vi "Start Video.vi"(4 "AVI Path":path, 5 "Offset":cluster{"Ch1":u8, "Ch2":u8}, 6 "Save Movie?":bool, 7 "Gain(dB)":cluster{"Ch1":dbl, "Ch2":dbl}, 8 "error in":errorcluster, 9 "Frame Rate(Hz)":cluster{"AVI FR":i32, "Camera Fr":u16}={"AVI FR"=30, "Camera Fr"=0} {"AVI FR" min=2 max=3000 step=1}, 10 "Trigger Type":enum16{"Internal", "External"}(ring)=enum."External", 11 "Region of interest":i32[](array[numeric])) -> (0 "error out":errorcluster, 1 "Frame Buffers Out":T2[](array[typedef]), 2 "Avi Refnum":T1, 3 "IMAQ Session Out":refnum<k11>)   [LabVIEW 2013]
uses:
  <vilib>/vision/Image Controls.llb/IMAQ Image.ctl
  <vilib>/vision/Avi1.llb/AviRefnum.ctl
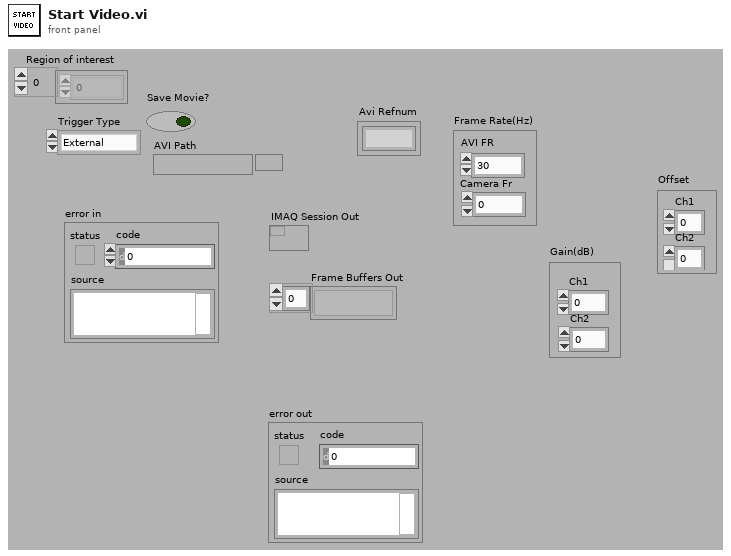
[diagram p1: front panel]
types:
  T1 = typedef "AviRefnum.ctl" = refnum<k1>
  T2 = typedef "IMAQ Image.ctl" = refnum<image>
  T3 = typedef "Image Type" = u32
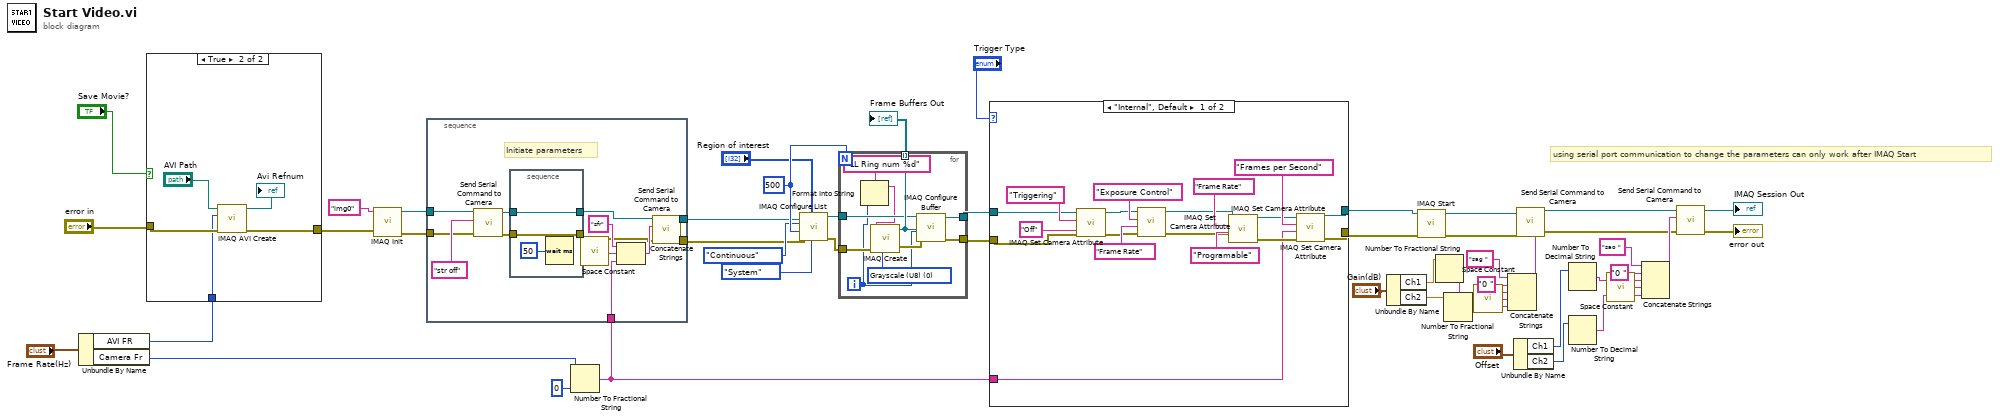
[diagram p0: block diagram]
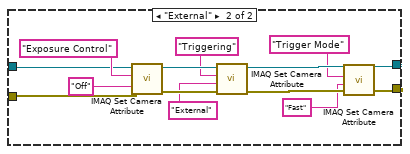
[diagram p3: hidden frame]
diagram:
  w49 = 500 ("Number of buffers")
  # "using serial port communication to change the parameters can only work after IMAQ Start"
  n1 = Unbundle By Name("Frame Rate(Hz)") -> ("AVI FR"=w27:i32, "Camera Fr"=w26:u16)
  n2 = case shown="True" "Save Movie?" {
    tunnel: "error in" -> [w50 w55]
    tunnel: [w50 w54] -> w40
    tunnel: w27 -> [_ w51]
    frame False {
    }
    frame True {
      n3 = call "IMAQ AVI Create"("error in (no error)"=w55, "Frames Per Second"=w51, "AVI Path"="AVI Path") -> ("error out"=w54:errorcluster, "Avi Refnum"=→"Avi Refnum":T1)  [unwired: 7 in]
    }
  }
  n4 = call <vilib>:"IMAQ Init.vi"("error in (no error)"=w40, "Interface Name"="img0") -> ("error out"=w35:errorcluster, "IMAQ Session Out"=w36:refnum<k11>)  [unwired: 8 in]
  n5 = Number To Fractional String(number=w26, precision (6)=i16 0) -> (F-format string=w31:string)  [unwired: 2 in]
  n6 = stacked-sequence {
    tunnel: w36 -> [w60]
    tunnel: w35 -> [w59]
    tunnel: [w58] -> w34
    tunnel: [w57] -> w33
    tunnel: w31 -> [w56]
    frame #0 {
      # "Initiate parameters"
      n7 = call "Send Serial Command to Camera.vi"("error in (no error)"=w59, "String to write"="str off", "IMAQ Session In"=w60) -> ("error out"=w62:errorcluster, "IMAQ Session Out"=w64:refnum<k11>)  [unwired: 5 in, 2 out]
      n8 = stacked-sequence {
        tunnel: w64 -> [w71]
        tunnel: [w71] -> w63
        tunnel: w62 -> [w70]
        tunnel: [w70] -> w61
        frame #0 {
          n9 = Wait (ms)(milliseconds to wait=u32 50) -> ()  [unwired: 1 out]
        }
      }
      n10 = call <vilib>:"Space Constant.vi"() -> ("String"=w66:string)
      n11 = Concatenate Strings("sfr" ("string"), w66, w56) -> (w65:string)
      n12 = call "Send Serial Command to Camera.vi"("error in (no error)"=w61, "String to write"=w65, "IMAQ Session In"=w63) -> ("error out"=w57:errorcluster, "IMAQ Session Out"=w58:refnum<k11>)  [unwired: 5 in, 2 out]
    }
  }
  n13 = call <vilib>:"IMAQ Configure List.vi"("Memory Location"=enum16{"System", "Onboard"}."System", "Region of interest"="Region of interest", "error in (no error)"=w33, "Number of buffers"=w49, "Continuous?"=enum16{"One-Shot", "Continuous"}."Continuous" ("Continuous ?"), "IMAQ Session In"=w34) -> ("error out"=w42:errorcluster, "IMAQ Session Out"=w43:refnum<k11>)  [unwired: 4 in]
  n14 = for {
    N: w49 -> [_]
    tunnel: [w81] -> w38
    tunnel: [w73] -> w37
    tunnel: w42 -> [w80]
    tunnel: w43 -> [w77]
    tunnel: [w78] -> w47 mode=indexing
    i -> [w74]
    w72 = T3 0 items=["Grayscale (U8)", "Grayscale (I16)", "Grayscale (SGL)", "Complex (CSG)", "RGB (U32)", "HSL (U32)", "RGB (U64)"] ("Image Type")
    n15 = Format Into String(format string="LL Ring num %d", w74) -> (resulting string=w76:string)  [unwired: 2 in, 1 out]
    n16 = call "IMAQ Create"("Image Name"=w76, "Image Type"=w72, "error in (no error)"=w80) -> ("New Image"=w78:T2, "error out"=w79:errorcluster)  [unwired: 2 in]
    n17 = call <vilib>:"IMAQ Configure Buffer.vi"("error in (no error)"=w79, "Buffer Number"=w74, "Image In"=w78, "IMAQ Session In"=w77) -> ("error out"=w73:errorcluster, "IMAQ Session Out"=w81:refnum<k11>)  [unwired: 6 in]
  }
  "Frame Buffers Out" <- w47
  n18 = case shown="\"Internal\", Default" "Trigger Type" {
    tunnel: w38 -> [w86 w103]
    tunnel: w37 -> [w85 w102]
    tunnel: w31 -> [w84 _]
    tunnel: [w83 w100] -> w30
    tunnel: [w82 w101] -> w29
    frame "Internal", Default {
      n19 = call <vilib>:"IMAQ Set Camera Attribute.vi"("error in (no error)"=w85, "Attribute Value"="Off", "Camera Attribute"="Triggering", "IMAQ Session In"=w86) -> ("error out"=w91:errorcluster, "IMAQ Session Out"=w93:refnum<k11>)  [unwired: 4 in]
      n20 = call <vilib>:"IMAQ Set Camera Attribute.vi"("error in (no error)"=w91, "Attribute Value"="Frame Rate", "Camera Attribute"="Exposure Control", "IMAQ Session In"=w93) -> ("error out"=w92:errorcluster, "IMAQ Session Out"=w94:refnum<k11>)  [unwired: 4 in]
      n21 = call <vilib>:"IMAQ Set Camera Attribute.vi"("error in (no error)"=w92, "Attribute Value"="Programable", "Camera Attribute"="Frame Rate", "IMAQ Session In"=w94) -> ("error out"=w90:errorcluster, "IMAQ Session Out"=w89:refnum<k11>)  [unwired: 4 in]
      n22 = call <vilib>:"IMAQ Set Camera Attribute.vi"("error in (no error)"=w90, "Attribute Value"=w84, "Camera Attribute"="Frames per Second", "IMAQ Session In"=w89) -> ("error out"=w82:errorcluster, "IMAQ Session Out"=w83:refnum<k11>)  [unwired: 4 in]
    }
    frame "External" {
      n23 = call <vilib>:"IMAQ Set Camera Attribute.vi"("error in (no error)"=w102, "Attribute Value"="Off", "Camera Attribute"="Exposure Control", "IMAQ Session In"=w103) -> ("error out"=w111:errorcluster, "IMAQ Session Out"=w109:refnum<k11>)  [unwired: 4 in]
      n24 = call <vilib>:"IMAQ Set Camera Attribute.vi"("error in (no error)"=w111, "Attribute Value"="External", "Camera Attribute"="Triggering", "IMAQ Session In"=w109) -> ("error out"=w110:errorcluster, "IMAQ Session Out"=w108:refnum<k11>)  [unwired: 4 in]
      n25 = call <vilib>:"IMAQ Set Camera Attribute.vi"("error in (no error)"=w110, "Attribute Value"="Fast", "Camera Attribute"="Trigger Mode", "IMAQ Session In"=w108) -> ("error out"=w101:errorcluster, "IMAQ Session Out"=w100:refnum<k11>)  [unwired: 4 in]
    }
  }
  n26 = Unbundle By Name("Gain(dB)") -> ("Ch1"=w15:dbl, "Ch2"=w14:dbl)
  n27 = call <vilib>:"IMAQ Start.vi"("error in (no error)"=w29, "IMAQ Session In"=w30) -> ("error out"=w16:errorcluster, "IMAQ Session Out"=w17:refnum<k11>)  [unwired: 8 in]
  n28 = Number To Fractional String(number=w15) -> (F-format string=w19:string)  [unwired: 3 in]
  n29 = Number To Fractional String(number=w14) -> (F-format string=w21:string)  [unwired: 3 in]
  n30 = call <vilib>:"Space Constant.vi"() -> ("String"=w20:string)
  n31 = Concatenate Strings("sag " ("String to write"), "0 " ("string"), w19, w20, w21) -> (w18:string)
  n32 = Unbundle By Name("Offset") -> ("Ch1"=w5:u8, "Ch2"=w4:u8)
  n33 = call "Send Serial Command to Camera.vi"("error in (no error)"=w16, "String to write"=w18, "IMAQ Session In"=w17) -> ("error out"=w6:errorcluster, "IMAQ Session Out"=w7:refnum<k11>)  [unwired: 5 in, 2 out]
  n34 = Number To Decimal String(number=w5) -> (decimal integer string=w9:string)  [unwired: 1 in]
  n35 = Number To Decimal String(number=w4) -> (decimal integer string=w8:string)  [unwired: 1 in]
  n36 = call <vilib>:"Space Constant.vi"() -> ("String"=w11:string)
  n37 = Concatenate Strings("sao " ("String to write"), "0 " ("string"), w9, w11, w8) -> (w10:string)
  n38 = call "Send Serial Command to Camera.vi"("error in (no error)"=w6, "String to write"=w10, "IMAQ Session In"=w7) -> ("error out"=→"error out":errorcluster, "IMAQ Session Out"=→"IMAQ Session Out":refnum<k11>)  [unwired: 5 in, 2 out]
